vi "Add Logging to Serial.vi"(8 "error in (no error)":errorcluster, 10 "Log Destination":refnum<class "Log.lvclass">, 11 "Serial":refnum<class "Serial.lvclass">) -> (0 "error out":errorcluster, 3 "Serial with Logging":refnum<class "Serial.lvclass">)   [LabVIEW 2020, in "Serial Logging Decorator.lvclass"]
uses:
  Serial Logging Decorator.lvclass
  Serial/Serial.lvclass/Serial.lvclass
  Log/Log.lvclass
  C:/git/astemes-lmock/sandbox/Examples/Serial/Serial.lvclass/Serial.lvclass
  Serial Logging Decorator.lvclass/Serial Logging Decorator.ctl
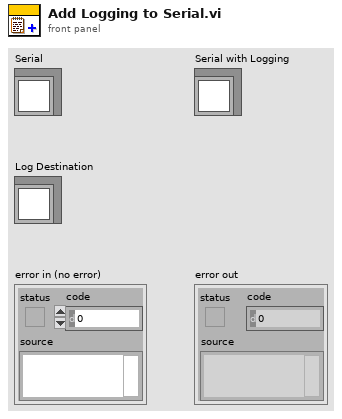
[diagram p1: front panel]
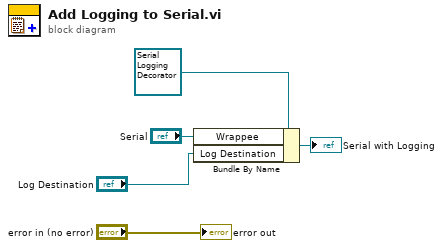
[diagram p0: block diagram]
diagram:
  n1 = Bundle By Name(cluster=refnum<class "Serial Logging Decorator.lvclass"> refnum ("Serial Logging Decorator.lvclass"), "Wrappee"="Serial", "Log Destination"="Log Destination") -> (→"Serial with Logging":refnum<class "Serial Logging Decorator.lvclass">)
  "error out" <- "error in (no error)"
